vi "Handle Error.vi"(8 "error in (no error)":errorcluster, 11 "HardwareSetup_modle001:HardwareSetup_modle001":refnum<class "HardwareSetup_model001.lvclass">) -> (0 "error out":errorcluster, 2 "stop actor?":bool=TRUE, 3 "HardwareSetup_modle001:HardwareSetup_modle001":refnum<class "HardwareSetup_model001.lvclass">)   [LabVIEW 2019, in "HardwareSetup_model001.lvlib" / "HardwareSetup_model001.lvclass"]
uses:
  HardwareSetup_model001.lvclass
  SystemSetup/SystemSetup/SystemSetup.lvclass
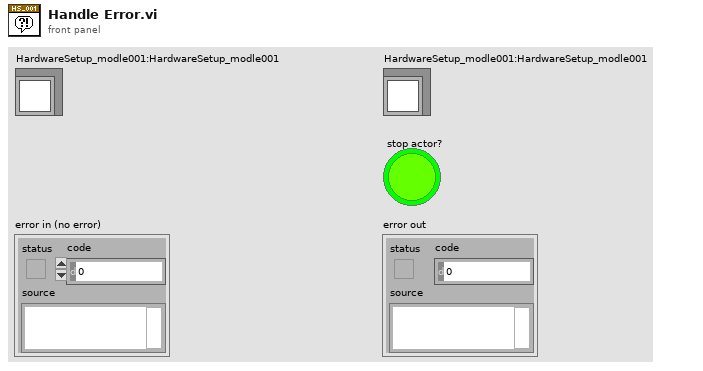
[diagram p1: front panel]
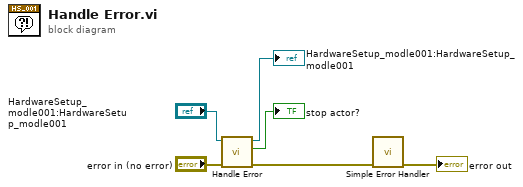
[diagram p0: block diagram]
diagram:
  n1 = call-parent "Handle Error.vi"("error in (no error)"="error in (no error)", "Actor in"="HardwareSetup_modle001:HardwareSetup_modle001") -> ("error out"=w6:errorcluster, "stop actor?"=→"stop actor?":bool, "Actor out"=→"HardwareSetup_modle001:HardwareSetup_modle001":refnum<class "HardwareSetup_model001.lvclass">)  [unwired: 7 in]
  n2 = call <vilib>:"Simple Error Handler.vi"("error in (no error)"=w6) -> ("error out"=→"error out":errorcluster)  [unwired: 4 in, 4 out]
